vi "DidInit.vi"(7 "Init?":bool, 8 "error in (no error)":errorcluster, 11 "ModuleAdmin In":refnum<class "ModuleAdmin.lvclass">) -> (0 "error out":errorcluster, 3 "ModuleAdmin Out":refnum<class "ModuleAdmin.lvclass">)   [LabVIEW 2018, in "ScopePlugins.lvlib"]
uses:
  ScopePlugins.lvlib
  <userlib>/NIST/ModuleAdminLib/ModuleAdmin/ModuleAdmin.lvclass
  ScopeShared/clEventType.ctl
  ScopeShared/clDidInit.ctl
  ScopeShared/ScopeShared.lvlib
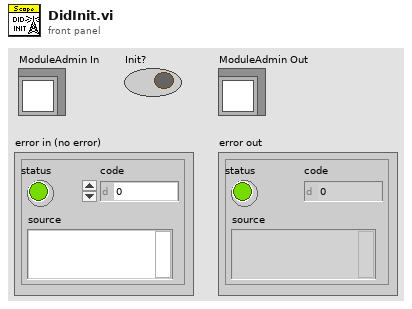
[diagram p1: front panel]
types:
  T1 = typedef "ScopeShared.lvlib/clDidInit.ctl" = cluster{"Init?":bool, "ModuleAdmin":refnum<class "ModuleAdmin.lvclass">}
  T2 = typedef "ScopeShared.lvlib/clEventType.ctl" = cluster{"ModuleID":i32, "Data":variant}
  T3 = typedef "ScopeShared.lvlib/clBroadcastEvents.ctl" = cluster{"DidInit":refnum<user-event>, "StatusUpdate":refnum<user-event>, "ErrorReport":refnum<user-event>, "DidStop":refnum<user-event>, "PathToINI":refnum<user-event>, "Handle":refnum<user-event>, "Model":refnum<user-event>, "Channels":refnum<user-event>, "Acquisition":refnum<user-event>, "Trigger":refnum<user-event>, "ExtAcquisition":refnum<user-event>, "Waveform":refnum<user-event>}
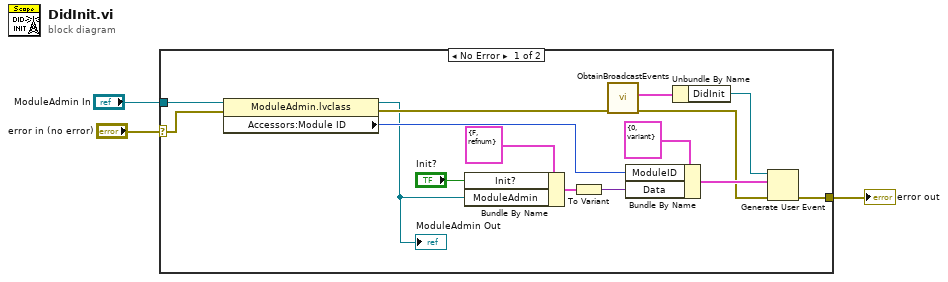
[diagram p0: block diagram]
diagram:
  n1 = case shown="No Error" "error in (no error)" {
    selector: "error in (no error)" -> [w7 w19]
    tunnel: [w11 w19] -> w3
    tunnel: "ModuleAdmin In" -> [w8 _]
    frame No Error {
      n2 = property class="ModuleAdmin.lvclass"(reference=w8, error in=w7) -> (reference out=w4:refnum<class "ModuleAdmin.lvclass">, error out=w6:errorcluster, "Accessors:Module ID"=w9:i32)
      "ModuleAdmin Out" <- w4
      n3 = Bundle By Name(cluster=T1 {"Init?"=FALSE, "ModuleAdmin"=refnum} ("clDidInit"), "Init?"="Init?", "ModuleAdmin"=w4) -> (w16:T1)
      n4 = To Variant(anything=w16) -> (Variant=w13:variant)
      n5 = call "ObtainBroadcastEvents.vi"("error in (no error)"=w6) -> ("error out"=w5:errorcluster, "clBroadcastEvents"=w17:T3)  [unwired: 9 in]
      n6 = Bundle By Name(cluster=T2 {"ModuleID"=0, "Data"=variant} ("clBroadcast"), "ModuleID"=w9, "Data"=w13) -> (w12:T2)
      n7 = Unbundle By Name(w17) -> ("DidInit"=w15:refnum<user-event>)
      n8 = Generate User Event(user event=w15, event data cluster=w12, error in=w5) -> (error out=w11:errorcluster)  [unwired: 1 in, 1 out]
    }
    frame Error {
    }
  }
  "error out" <- w3
